vi "InitDataSets.vi"(8 "error in (no error)":errorcluster, 10 "registry":T3, 11 "dataevent":T1) -> (0 "error out":errorcluster, 2 "datasetIds":variant, 3 "datasets":T7[](array[typedef]))   [LabVIEW 2017, in "McsaDataEventCreator.lvlib"]
uses:
  <vilib>/addons/InsightCM/Devices/Shared/Mcsa/McsaDataEventCreator/McsaDataEventCreator.lvlib
  <vilib>/addons/InsightCM/Devices/Shared/Common/DataEvent/controls/DataSet.ctl
  <vilib>/addons/InsightCM/MessageBus/Base/controls/DataSetMetadata.ctl
  <vilib>/addons/InsightCM/MessageBus/Base/controls/KeyValuePair.ctl
  <vilib>/addons/InsightCM/Devices/Shared/Mcsa/McsaDataEventCreator/controls/DataGroupRegistry.ctl
  <vilib>/addons/InsightCM/Devices/Shared/Mcsa/McsaDataEventCreator/controls/Registry_DataSet.ctl
  <vilib>/addons/InsightCM/Devices/Shared/Mcsa/McsaDataEventCreator/controls/DataSetType.ctl
  <vilib>/addons/InsightCM/Devices/Shared/Common/DataEventCreator/controls/Registry_Trend.ctl
  <vilib>/addons/InsightCM/MessageBus/Base/controls/DataEvent.ctl
  <vilib>/addons/InsightCM/Devices/Shared/Common/DataEvent/DataEvent.lvlib
  <vilib>/addons/InsightCM/SRP/SRP.lvlib
  <vilib>/addons/InsightCM/Utilities/PropertyHelpers/PropertyHelpers.lvlib
  <vilib>/addons/InsightCM/Devices/Shared/Common/DataEventCreator/DataEventCreator.lvlib
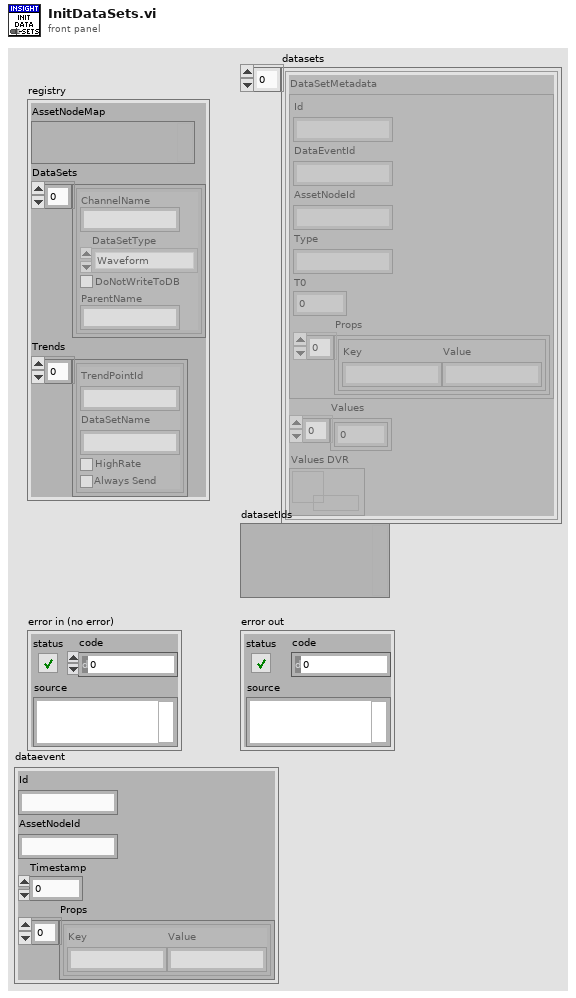
[diagram p1: front panel]
types:
  T1 = typedef "DataEvent.ctl" = cluster{"Id":string, "AssetNodeId":string, "Timestamp":i64, "Props":T2[]}
  T2 = typedef "KeyValuePair.ctl" = cluster{"Key":string, "Value":string}
  T3 = typedef "McsaDataEventCreator.lvlib/DataGroupRegistry.ctl" = cluster{"AssetNodeMap":variant, "DataSets":T4[], "Trends":T6[]}
  T4 = typedef "McsaDataEventCreator.lvlib/Registry_DataSet.ctl" = cluster{"ChannelName":string, "DataSetType":T5, "DoNotWriteToDB":bool, "ParentName":string}
  T5 = typedef "McsaDataEventCreator.lvlib/DataSetType.ctl" = enum16{"Waveform", "MCSAFFT", "TorqueWFM"}
  T6 = typedef "DataEventCreator.lvlib/Registry_Trend.ctl" = cluster{"TrendPointId":string, "DataSetName":string, "HighRate":bool, "Always Send":bool}
  T7 = typedef "DataEvent.lvlib/DataSet.ctl" = cluster{"DataSetMetadata":T8, "Values":sgl[], "Values DVR":refnum<data-value>}
  T8 = typedef "DataSetMetadata.ctl" = cluster{"Id":string, "DataEventId":string, "AssetNodeId":string, "Type":string, "T0":i64, "Props":T2[]}
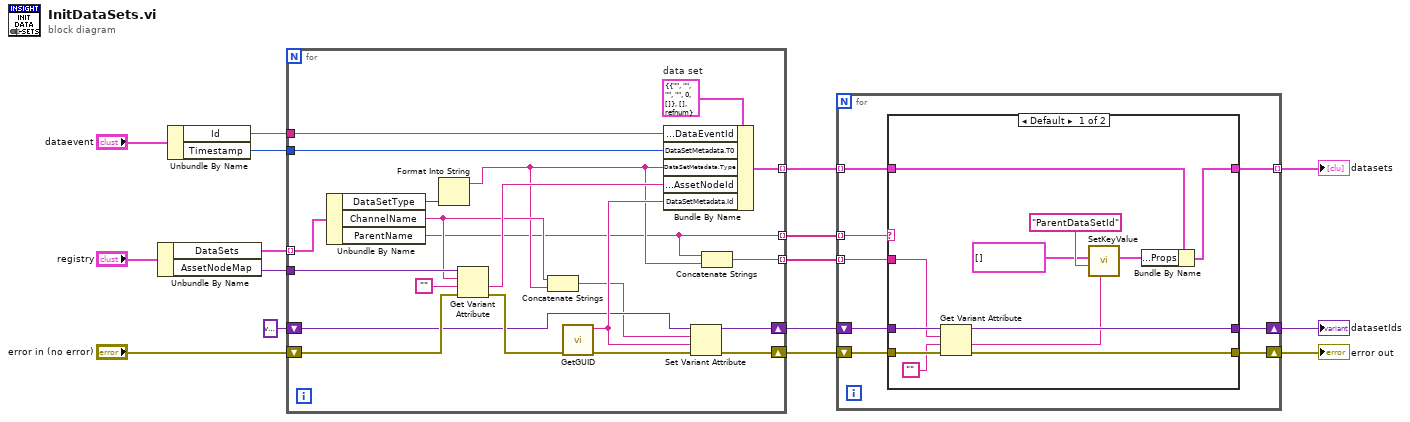
[diagram p0: block diagram]
diagram:
  n1 = Unbundle By Name("registry") -> ("DataSets"=w6:T4[], "AssetNodeMap"=w8:variant)
  n2 = Unbundle By Name("dataevent") -> ("Id"=w3:string, "Timestamp"=w2:i64)
  n3 = for {
    tunnel: w6 -> [w25] mode=indexing
    tunnel: w8 -> [w31]
    shift-right: [w36] -> w11
    shift-left: variant -> [w24]
    shift-right: [w35] -> w12
    shift-left: "error in (no error)" -> [w33]
    tunnel: [w27] -> w10 mode=indexing
    tunnel: [w19] -> w15 mode=indexing
    tunnel: w3 -> [w23]
    tunnel: w2 -> [w22]
    tunnel: [w17] -> w1 mode=indexing
    w29 = T7 {"DataSetMetadata"={"Id"="", "DataEventId"="", "AssetNodeId"="", "Type"="", "T0"=0, "Props"=[]}, "Values"=[], "Values DVR"=refnum}  # data set
    n4 = Unbundle By Name(w25) -> ("DataSetType"=w34:T5, "ChannelName"=w21:string, "ParentName"=w17:string)
    n5 = Format Into String(w34) -> (resulting string=w18:string)  [unwired: 3 in, 1 out]
    n6 = Get Variant Attribute(Variant=w31, name=w21, default value (empty Variant)="", error in=w33) -> (value=w28:string, error out=w32:errorcluster)  [unwired: 2 out]
    n7 = Concatenate Strings(w21, w18) -> (w20:string)
    n8 = call <vilib>:"GetGUID.vi"("error in (no error)"=w32) -> ("error out"=w37:errorcluster, "GUID"=w26:string)  [unwired: 9 in]
    n9 = Bundle By Name(cluster=w29, "DataSetMetadata.DataEventId"=w23, "DataSetMetadata.T0"=w22, "DataSetMetadata.Type"=w18, "DataSetMetadata.AssetNodeId"=w28, "DataSetMetadata.Id"=w26) -> (w27:T7)
    n10 = Set Variant Attribute(Variant=w24, name=w20, value=w26, error in=w37) -> (Variant out=w36:variant, error out=w35:errorcluster)  [unwired: 1 out]
    n11 = Concatenate Strings(w17, w18) -> (w19:string)
  }
  n12 = for {
    tunnel: w10 -> [w45] mode=indexing
    shift-right: [w42] -> w13
    shift-left: w11 -> [w44]
    shift-right: [w41] -> w14
    shift-left: w12 -> [w43]
    tunnel: w15 -> [w39] mode=indexing
    tunnel: [w40] -> w16 mode=indexing
    tunnel: w1 -> [w38] mode=indexing
    n13 = case shown="Default" w38 {
      tunnel: w45 -> [w57 w58]
      tunnel: w44 -> [w56 w60]
      tunnel: w43 -> [w55 w59]
      tunnel: [w52 w60] -> w42
      tunnel: [w51 w59] -> w41
      tunnel: [w48 w58] -> w40
      tunnel: w39 -> [w46 _]
      frame Default {
        n14 = Get Variant Attribute(Variant=w56, name=w46, default value (empty Variant)="", error in=w55) -> (duplicate Variant=w52:variant, value=w50:string, error out=w51:errorcluster)  [unwired: 1 out]
        n15 = call <vilib>:"SetKeyValue.vi"("value"=w50, "key"="ParentDataSetId", "key value pairs"=T2[] []) -> ("key value pairs out"=w53:T2[])  [unwired: 8 in]
        n16 = Bundle By Name(cluster=w57, "DataSetMetadata.Props"=w53) -> (w48:T7)
      }
      frame "" {
      }
    }
  }
  "datasets" <- w16
  "error out" <- w14
  "datasetIds" <- w13
